vi "Get-Elapsed-Time.vi"() -> (3 "ElapsedTime":dbl)   [LabVIEW 2019]
uses:
  <vilib>/Rock Robotics/WPI/ThirdParty/JAS_Junk/TrajLib/Trajectory_Library.lvlib
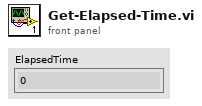
[diagram p1: front panel]
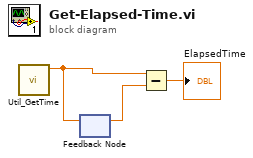
[diagram p0: block diagram]
diagram:
  n1 = call <vilib>:"Util_GetTime.vi"() -> ("FPGA_Time_Seconds"=w2:dbl)  [unwired: 10 in, 1 out]
  n2 = feedback-in #1(w2) -> ()
  n3 = feedback #1() -> (w1:dbl)  [unwired: 1 in]
  n4 = Subtract(x=w2, y=w1) -> (x-y=→"ElapsedTime":dbl)
